vi "action.vi"(0 "NInstrSim_ReadStatus":refnum<class "NInstrSim_ReadStatus.lvclass">, 2 "HGF_Visitable":refnum<class "HGF_Visitable.lvclass">, 5 "error in (no error)":errorcluster) -> (14 "dup NInstrSim_ReadStatus":refnum<class "NInstrSim_ReadStatus.lvclass">, 16 "dup HGF_Visitable":refnum<class "HGF_Visitable.lvclass">, 19 "error out":errorcluster)   [LabVIEW 2009, in "HB_Device_Examples.lvlib" / "NInstrSim_ReadStatus.lvclass"]
doc: "This is a dynamic dispatch VI that is called from Visitor.visit(). It will call member VIs of Visitable to perform the requested action which means: calling public methods of Visitable child class.\n\n<B>Hint:</B> This method is abstract and need to be implemented by child classes."
uses:
  NInstrSim_ReadStatus.lvclass
  lib.lib/HGF_LVC/HGF_BaseClasses/HGF_Visitable/HGF_Visitable.lvclass
  NInstrSim.lvclass
  NInstrSim_ReadStatus.lvclass/NInstrSim_ReadStatus.ctl
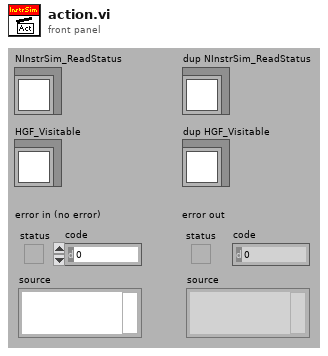
[diagram p1: front panel]
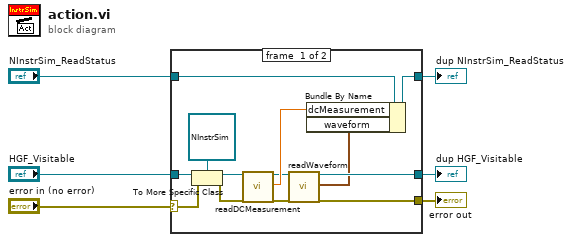
[diagram p0: block diagram]
diagram:
  n1 = case shown="No Error" "error in (no error)" {
    selector: "error in (no error)" -> [w17 w20]
    tunnel: "NInstrSim_ReadStatus" -> [w16 w22]
    tunnel: "HGF_Visitable" -> [w19 w21]
    tunnel: [w14 w21] -> w4
    tunnel: [w13 w20] -> w3
    tunnel: [w15 w22] -> w1
    frame #0 {
      n2 = To More Specific Class(target class=refnum<class "NInstrSim.lvclass"> refnum ("HB_HGF_Test.lvlib:NInstrSim.lvclass"), reference=w19, error in=w17) -> (specific class reference=w9:refnum<class "NInstrSim.lvclass">, error out=w10:errorcluster)
      n3 = call "readDCMeasurement.vi"("NInstrSim"=w9, "error in (no error)"=w10) -> ("dup NInstrSim"=w7:refnum<class "NInstrSim.lvclass">, "DC Measurement"=w8:dbl, "error out"=w11:errorcluster)  [unwired: 15 out]
      n4 = call "readWaveform.vi"("NInstrSim"=w7, "error in (no error)"=w11) -> ("dup NInstrSim"=w14:refnum<class "NInstrSim.lvclass">, "Waveform"=w12:waveform(dbl), "error out"=w13:errorcluster)  [unwired: 15 out]
      n5 = Bundle By Name(cluster=w16, "dcMeasurement"=w8, "waveform"=w12) -> (w15:refnum<class "NInstrSim_ReadStatus.lvclass">)
    }
    frame #1 {
    }
  }
  "error out" <- w3
  "dup NInstrSim_ReadStatus" <- w1
  "dup HGF_Visitable" <- w4
